vi "Insert Main SubPanel.vi"(8 "error in (no error)":errorcluster, 9 "ActorQName":string, 10 "CalleeActorVI Ref":refnum<vi>, 11 "CallActorCenter in":refnum<class "CallActorCenter.lvclass">) -> (0 "error out":errorcluster, 3 "CallActorCenter out":refnum<class "CallActorCenter.lvclass">)   [LabVIEW 2021, in "CallActorCenter.lvclass"]
uses:
  CallActorCenter.lvclass
  CallActorCenter.lvclass/CallActorCenter.ctl
  <vilib>/ActorFramework/Actor/Actor.lvclass
  <userlib>/John_Lib/Interfaces/InsertMainSubPanel Messages/Insert Main SubPanel Msg/Insert Main SubPanel Msg.lvclass
  C:/Program Files (x86)/National Instruments/LabVIEW 2021/user.lib/John_Lib/AbstractActorTemplate/AbstractActorTemplate/UIActorTop.lvclass
  C:/Program Files (x86)/National Instruments/LabVIEW 2021/vi.lib/ActorFramework/Actor/Actor.lvclass
  C:/Program Files (x86)/National Instruments/LabVIEW 2021/project/Create Actor from Template/_CallActorCenter/CallActorCenter.lvclass
  C:/Program Files (x86)/National Instruments/LabVIEW 2021/user.lib/John_Lib/Interfaces/InsertLeftSubPanel/InsertLeftSubPanel.lvclass
  C:/Program Files (x86)/National Instruments/LabVIEW 2021/user.lib/John_Lib/Interfaces/InsertMainSubPanel/InsertMainSubPanel.lvclass
  C:/Program Files (x86)/National Instruments/LabVIEW 2021/user.lib/John_Lib/Interfaces/InsertRightSubPanel/InsertRightSubPanel.lvclass
  C:/Program Files (x86)/National Instruments/LabVIEW 2021/user.lib/John_Lib/Interfaces/FrontPanel Save Image/FrontPanel Save Image.lvclass
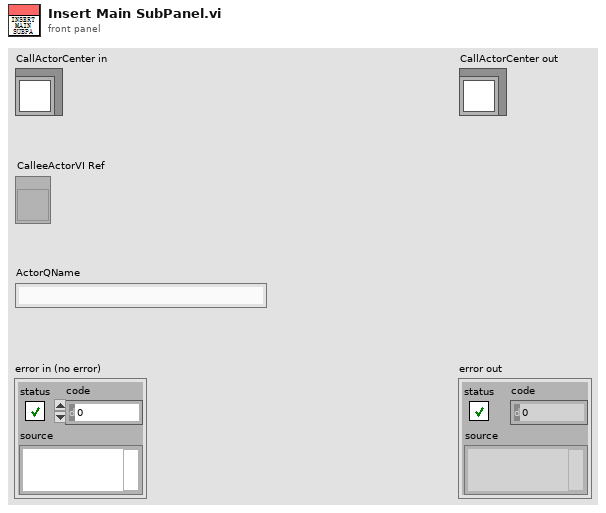
[diagram p1: front panel]
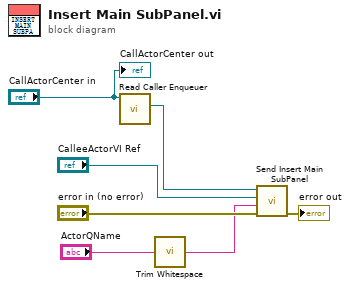
[diagram p0: block diagram]
diagram:
  n1 = call <vilib>:"Read Caller Enqueuer.vi"("Actor"="CallActorCenter in") -> ("Caller Enqueuer"=w6:refnum<class "Message Enqueuer.lvclass">)  [unwired: 10 in]
  n2 = call <vilib>:"Trim Whitespace.vi"("string"="ActorQName") -> ("trimmed string"=w1:string)  [unwired: 1 in]
  n3 = call <userlib>:"Send Insert Main SubPanel.vi"("error in (no error)"="error in (no error)", "ActorQName"=w1, "CalleeActorVI Ref"="CalleeActorVI Ref", "Message Enqueuer"=w6) -> ("error out"=→"error out":errorcluster)  [unwired: 6 in, 1 out]
  "CallActorCenter out" <- "CallActorCenter in"
